vi "Path for cust seq shots.vi"(4 "Diff Prefix?":bool=TRUE caption="Same Prefix", 6 "Index":u16, 8 "SubfolderName":string[](array[string])=["", "", "", "", "", ""], 9 "File Path Input":T1={"Filename Prefix"="MyData", "Extension"=enum."±Field", "Suffix"="", "Current Path"=path "/opticsmac/Users/Data"}) -> (3 "File Path output":T1={"Filename Prefix"="MyData", "Extension"=enum."±Field", "Suffix"="", "Current Path"=path "/opticsmac/Users/Data"})   [LabVIEW 2020]
uses:
  Globals and TypeDefs/Type Definitions.llb/FilePathParameter.ctt
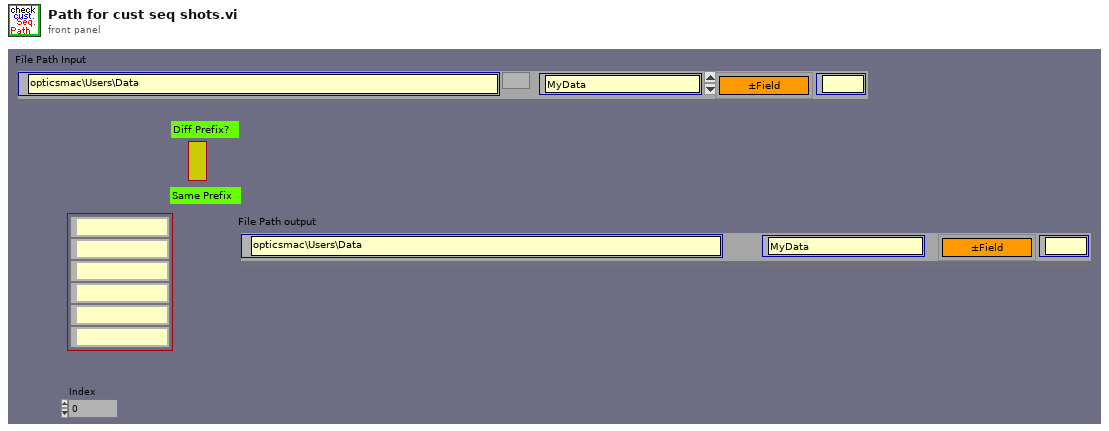
[diagram p1: front panel]
types:
  T1 = typedef "FilePathParameter.ctt" = cluster{"Filename Prefix":string, "Extension":enum16{"none", "\".001\",\".002\", ...", "001 (No dot)", "±Field", "pField nField", "Temperature", "Wavelength", "T(K)±H(T)", "(nm)T(K)±H(T)", "User Defined"}, "Suffix":string, "Current Path":path}
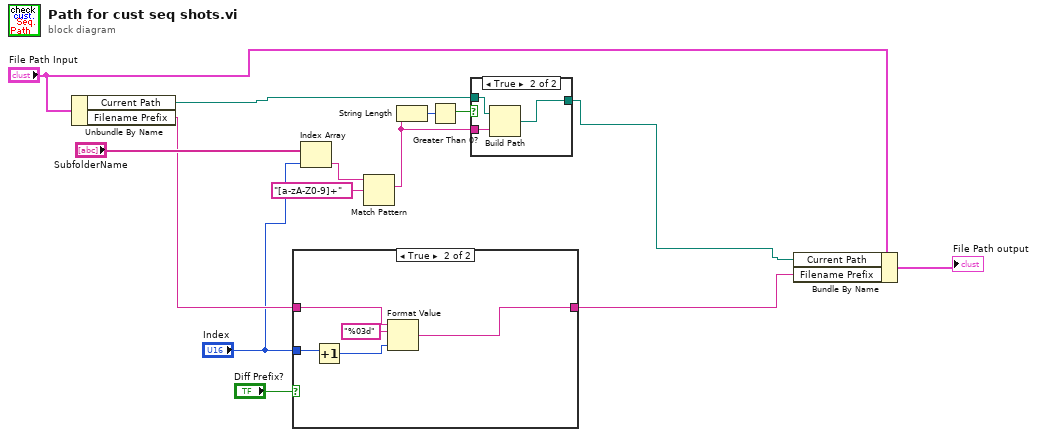
[diagram p0: block diagram]
diagram:
  n1 = Unbundle By Name("File Path Input") -> ("Current Path"=w9:path, "Filename Prefix"=w10:string)
  n2 = case shown="True" "Diff Prefix?" {
    tunnel: w10 -> [w15 w17]
    tunnel: [w15 w16] -> w14
    tunnel: "Index" -> [_ w20]
    frame False {
    }
    frame True {
      n3 = Increment(x=w20) -> (x+1=w18:u16)
      n4 = Format Value(string ("")=w17, format string="%03d", value (0)=w18) -> (output string=w16:string)
    }
  }
  n5 = Index Array(array="SubfolderName", index="Index") -> (element=w5:string)
  n6 = Match Pattern(string=w5, regular expression="[a-zA-Z0-9]+") -> (match substring=w1:string)  [unwired: 1 in, 3 out]
  n7 = String Length(string=w1) -> (length=w3:i32)
  n8 = Greater Than 0?(x=w3) -> (x > 0?=w2:bool)
  n9 = case shown="True" w2 {
    tunnel: w1 -> [_ w24]
    tunnel: w9 -> [w21 w23]
    tunnel: [w21 w22] -> w8
    frame False {
    }
    frame True {
      n10 = Build Path(base path=w23, name or relative path=w24) -> (appended path=w22:path)
    }
  }
  n11 = Bundle By Name(cluster="File Path Input", "Current Path"=w8, "Filename Prefix"=w14) -> (→"File Path output":T1)
